vi "NI6602.i attribute.vi"(0 "VI Refnum":refnum<vi>, 2 "CLASS.i attribute":T1, 3 "Action":T2(ring), 5 "error in (no error)":errorcluster) -> (14 "VI Refnum out":refnum<vi>, 16 "CLASS.i attribute out":T1, 19 "error out":errorcluster)   [LabVIEW 2014, in "NI6602.lvlib"]
doc: "This is a so-called functional global variable. It manages the access to a global variable in a thread-safe way. \n\nHere the attribute data of all instances of THIS class are stored. This is done for performance reasons.\n\nLicense Agreement for this software:\n\nCopyright (C)\nGesellschaft für Schwerionenforschung, GSI\nPlanckstr. 1\n64291 Darmstadt\nGermany\n\nContact: D.Beck@gsi.de \n\nThis program is free software; you can redistribute it and/or modify it under the terms of the GNU General Public License as published by the Free Software Foundation; either version 2 of the license, or (at your option) any later version.\n\nThis program is distributed in the hope that it will be useful, but WITHOUT ANY WARRANTY; without even the implied warranty of MERCHANTABILITY or FITNESS FOR A PARTICULAR PURPOSE. See the GNU General License for more details (http://www.gnu.org).\n\nGesellschaft für Schwerionenforschung, GSI\nPlanckstr. 1, 64291 Darmstadt, Germany\nFor all questions and ideas contact: M.Richter@gsi.de, H.Brand@gsi.de or D.Beck@gsi.de.\nLast update: 17-JUN-2004"
uses:
  NI6602.lvlib
  NI6602.i attribute.ctl
  CS_Core/CSSystem/CoreDefs/CoreDefs.error_type.ctl
  CS_Core/CSSystem/CoreLib/CoreLib.lvlib
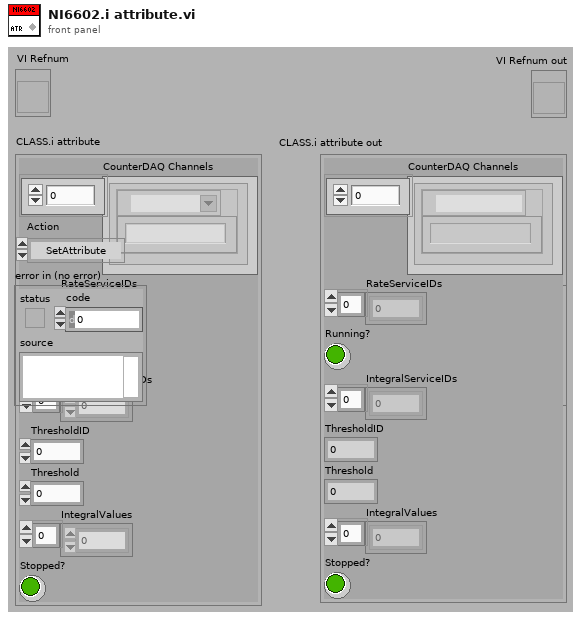
[diagram p1: front panel]
types:
  T1 = typedef "NI6602.lvlib/NI6602.i attribute.ctl" = cluster{"CounterDAQ Channels":cluster{"task":refnum<k21>, "Channel Name":string}[], "RateServiceIDs":i32[], "Running?":bool, "IntegralServiceIDs":i32[], "ThresholdID":i32, "Threshold":dbl, "IntegralValues":dbl[], "Stopped?":bool}
  T2 = enum16{"SetAttribute", "GetAttribute", "CreateAttribute", "DestroyAttribute", "DestroyAllAtributes"}
  T3 = typedef "CoreDefs.error_type.ctl" = enum16{"no error", "can't load process", "can't unload process", "process does not exist", "can't install process", "can't remove process", "unknown function", "time out", "can't execute function", "duplicate queue name", "super not found", "caller queue invalid", "can't ping process", "unknown error", "VISA Error", "VISA timeout", "GPIB timeout", "GPIB error", "communication error", "data type mismatch", "can't read data from OPC server", "can't write data to OPC server", "OET error", "function not implemented", "process already exists", "invalid Shared Variable name", "error writing Shared Variable", "error reading Shared Variable", "invalid client name", "corrupt database", "unknown class", "call not authorized", "parameter out of range", "OET timeout: can't get data to modify", "invalid queue name", "requested operation incompatible with current state", "event undefined", "event disabled", "state undefined", "caller is not a friend", "EventBuilder: bad eventID", "EventBuilder: no DAQ devices", "a thread must not stop itself", "UNUSED ELEMENT4", "DiscArchiver: eventData incomplete", "DiscArchiver: eventData does not belong to run", "DiscArchiver: can't open file", "DiscArchiver: can't write to file", "DiscArchiver: available disc space low", "can't acquire semaphore", "error reading data from database", "notifier object is not existing", "can't register process", "can't unregister process", "illegal event type", "object disabled", "object already exists", "can't change state", "Instrument not found", "no connection to remote node", "invalid reference", "N/A", "UNUSED ELEMENT 1", "element not found", "illegal TCP/IP connection detected", "object does not exist", "invalid access ID", "unknown CS system", "invalid privilige", "unsupported data type", "unsupported server type", "IO server already exists", "Shared Variable already exists"}
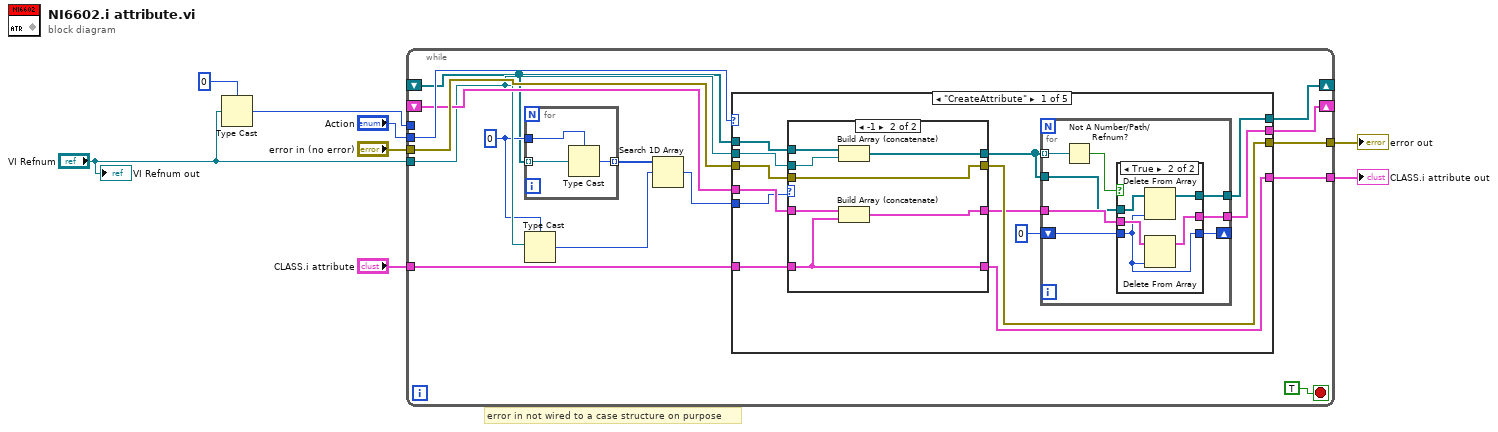
[diagram p0: block diagram]
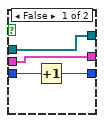
[diagram p2: hidden frame]
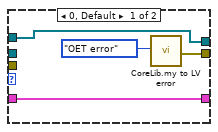
[diagram p3: hidden frame]
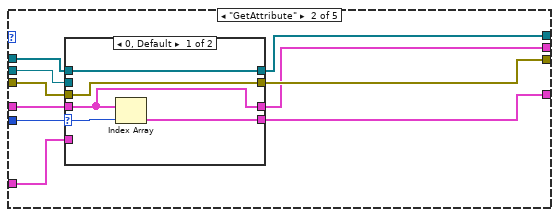
[diagram p4: hidden frame]
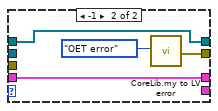
[diagram p5: hidden frame]
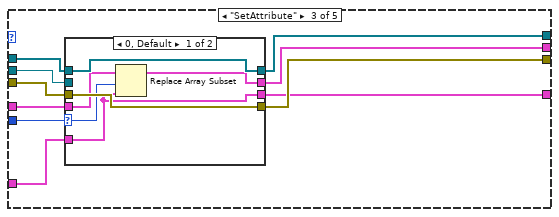
[diagram p6: hidden frame]
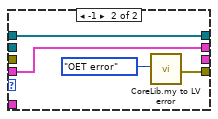
[diagram p7: hidden frame]
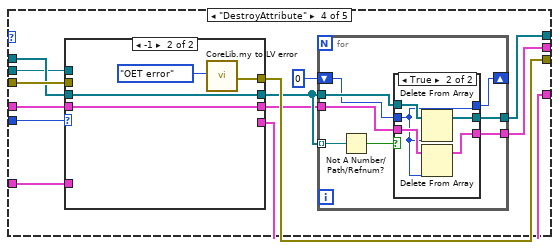
[diagram p8: hidden frame]
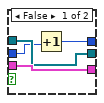
[diagram p9: hidden frame]
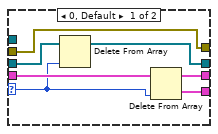
[diagram p10: hidden frame]
diagram:
  # "error in not wired to a case structure on purpose"
  n1 = Type Cast(type=0, x="VI Refnum") -> (*(type *) &x=w2:i32)
  n2 = while {
    shift-right: [w17] -> _
    shift-left: _ -> [w18]
    tunnel: "Action" -> [w22]
    shift-right: [w19] -> _
    shift-left: _ -> [w9]
    tunnel: w2 -> [_]
    tunnel: "error in (no error)" -> [w21]
    tunnel: [w20] -> w6
    tunnel: "CLASS.i attribute" -> [w16]
    tunnel: [w14] -> w4
    tunnel: "VI Refnum" -> [w12]
    stop <- TRUE stop-if-true
    w11 = 0
    n3 = for {
      tunnel: w11 -> [w26]
      tunnel: [w25] -> w10 mode=indexing
      tunnel: w9 -> [w24] mode=indexing
      n4 = Type Cast(type=w26, x=w24) -> (*(type *) &x=w25:i32)
    }
    n5 = Type Cast(type=w11, x=w12) -> (*(type *) &x=w13:i32)
    n6 = Search 1D Array(1D array=w10, element=w13) -> (index of element=w15:i32)  [unwired: 1 in]
    n7 = case shown="\"CreateAttribute\"" w22 {
      tunnel: w9 -> [w37 w75 w94 w117 _]
      tunnel: w12 -> [w36 w73 w92 w116 _]
      tunnel: w21 -> [w39 w77 w96 w119 w148]
      tunnel: [w38 w76 w95 w118 w148] -> w20
      tunnel: [w31 w74 w93 w111 _] -> w19
      tunnel: w18 -> [w35 w72 w91 w115 _]
      tunnel: [w30 w71 w90 w109 _] -> w17
      tunnel: w16 -> [w34 w70 w89 w114 _]
      tunnel: w15 -> [w33 w69 w88 w113 _]
      tunnel: [w27 w68 w87 w107 _] -> w14
      frame "CreateAttribute" {
        n8 = case shown="-1" w33 {
          tunnel: w39 -> [_ w67]
          tunnel: [w59 w67] -> w38
          tunnel: w37 -> [w58 w66]
          tunnel: [w58 w65] -> w29
          tunnel: w36 -> [_ w64]
          tunnel: w35 -> [w57 w63]
          tunnel: [w57 w62] -> w28
          tunnel: w34 -> [_ w61]
          tunnel: [_ w61] -> w27
          frame 0, Default {
            n9 = call "CoreLib.my to LV error.vi"("ErrorTypes"=CoreDefs.error_type."OET error") -> ("myErrorCluster"=w59:errorcluster)  [unwired: 17 in, 1 out]
          }
          frame -1 {
            n10 = Build Array (concatenate)(w66, w64) -> (w65:refnum<vi>[])
            n11 = Build Array (concatenate)(w63, w61) -> (w62:T1[])
          }
        }
        n12 = for {
          tunnel: w29 -> [w44]
          tunnel: [w43] -> w31
          tunnel: [w47] -> w30
          tunnel: w28 -> [w46]
          tunnel: w29 -> [w42] mode=indexing
          shift-right: [w41] -> _
          shift-left: 0 -> [w40]
          n13 = Not A Number/Path/Refnum?(number/path/refnum=w42) -> (NaN/Path/Refnum?=w45:bool)
          n14 = case shown="True" w45 {
            tunnel: [w51 w56] -> w47
            tunnel: w46 -> [w51 w55]
            tunnel: [w50 w53] -> w43
            tunnel: w44 -> [w50 w54]
            tunnel: w40 -> [w49 w52]
            tunnel: [w48 w52] -> w41
            frame False {
              n15 = Increment(x=w49) -> (x+1=w48:i32)
            }
            frame True {
              n16 = Delete From Array(array=w54, index=w52) -> (array with subset deleted=w53:refnum<vi>[])  [unwired: 1 in, 1 out]
              n17 = Delete From Array(array=w55, index=w52) -> (array with subset deleted=w56:T1[])  [unwired: 1 in, 1 out]
            }
          }
        }
      }
      frame "GetAttribute" {
        n18 = case shown="0, Default" w69 {
          selector: w69 -> [w80 _]
          tunnel: w77 -> [w82 _]
          tunnel: [w82 w85] -> w76
          tunnel: w75 -> [w81 w84]
          tunnel: [w81 w84] -> w74
          tunnel: w73 -> [_ _]
          tunnel: w72 -> [w79 w83]
          tunnel: [w79 w83] -> w71
          tunnel: w70 -> [_ _]
          tunnel: [w78 _] -> w68
          frame 0, Default {
            n19 = Index Array(array=w79, index=w80) -> (element=w78:T1)
          }
          frame -1 {
            n20 = call "CoreLib.my to LV error.vi"("ErrorTypes"=CoreDefs.error_type."OET error") -> ("myErrorCluster"=w85:errorcluster)  [unwired: 17 in, 1 out]
          }
        }
      }
      frame "SetAttribute" {
        n21 = case shown="0, Default" w88 {
          selector: w88 -> [w98 _]
          tunnel: w96 -> [w102 _]
          tunnel: [w102 w105] -> w95
          tunnel: w94 -> [w101 w104]
          tunnel: [w101 w104] -> w93
          tunnel: w92 -> [_ _]
          tunnel: w91 -> [w100 w103]
          tunnel: [w99 w103] -> w90
          tunnel: w89 -> [w97 _]
          tunnel: [w97 _] -> w87
          frame 0, Default {
            n22 = Replace Array Subset(array=w100, new element=w97, index=w98) -> (w99:T1[])
          }
          frame -1 {
            n23 = call "CoreLib.my to LV error.vi"("ErrorTypes"=CoreDefs.error_type."OET error") -> ("myErrorCluster"=w105:errorcluster)  [unwired: 17 in, 1 out]
          }
        }
      }
      frame "DestroyAttribute" {
        n24 = case shown="-1" w113 {
          selector: w113 -> [w139 _]
          tunnel: w119 -> [w143 _]
          tunnel: [w143 w146] -> w118
          tunnel: w117 -> [w142 w145]
          tunnel: [w141 w145] -> w110
          tunnel: w116 -> [_ _]
          tunnel: w115 -> [w140 w144]
          tunnel: [w138 w144] -> w108
          tunnel: w114 -> [_ _]
          tunnel: [w137 _] -> w107
          frame 0, Default {
            n25 = Delete From Array(array=w142, index=w139) -> (array with subset deleted=w141:refnum<vi>[])  [unwired: 1 in, 1 out]
            n26 = Delete From Array(array=w140, index=w139) -> (deleted portion=w137:T1, array with subset deleted=w138:T1[])  [unwired: 1 in]
          }
          frame -1 {
            n27 = call "CoreLib.my to LV error.vi"("ErrorTypes"=CoreDefs.error_type."OET error") -> ("myErrorCluster"=w146:errorcluster)  [unwired: 17 in, 1 out]
          }
        }
        n28 = for {
          tunnel: w110 -> [w124]
          tunnel: [w123] -> w111
          tunnel: [w127] -> w109
          tunnel: w108 -> [w126]
          tunnel: w110 -> [w122] mode=indexing
          shift-right: [w121] -> _
          shift-left: 0 -> [w120]
          n29 = Not A Number/Path/Refnum?(number/path/refnum=w122) -> (NaN/Path/Refnum?=w125:bool)
          n30 = case shown="True" w125 {
            tunnel: [w131 w136] -> w127
            tunnel: w126 -> [w131 w135]
            tunnel: [w130 w133] -> w123
            tunnel: w124 -> [w130 w134]
            tunnel: w120 -> [w129 w132]
            tunnel: [w128 w132] -> w121
            frame False {
              n31 = Increment(x=w129) -> (x+1=w128:i32)
            }
            frame True {
              n32 = Delete From Array(array=w134, index=w132) -> (array with subset deleted=w133:refnum<vi>[])  [unwired: 1 in, 1 out]
              n33 = Delete From Array(array=w135, index=w132) -> (array with subset deleted=w136:T1[])  [unwired: 1 in, 1 out]
            }
          }
        }
      }
      frame "DestroyAllAtributes" {
      }
    }
  }
  "error out" <- w6
  "CLASS.i attribute out" <- w4
  "VI Refnum out" <- "VI Refnum"
